vi "TIO SLIP Encode.vi"(2 "error in (no error)":errorcluster, 3 "String Input":string="\u00124VxÛ\u0000") -> (0 "error out":errorcluster, 1 "SLIP Output":string)   [LabVIEW 2017]
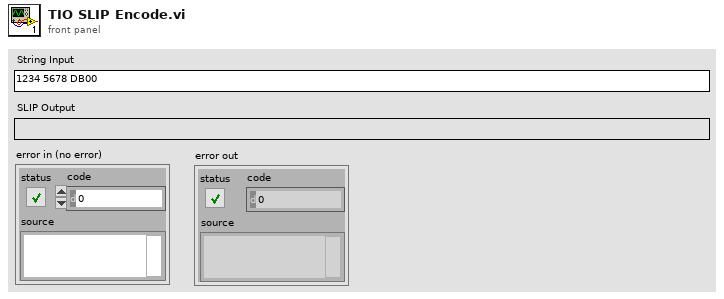
[diagram p1: front panel]
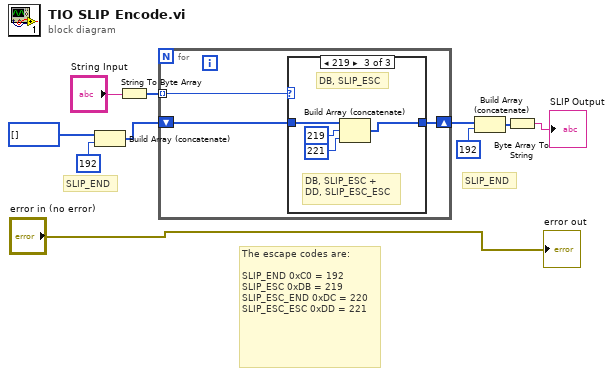
[diagram p0: block diagram]
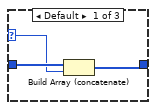
[diagram p2: hidden frame]
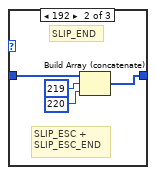
[diagram p3: hidden frame]
diagram:
  # "SLIP_END"
  # "SLIP_END"
  # "The escape codes are:\n\nSLIP_END\t0xC0 = 192\nSLIP_ESC\t0xDB = 219\nSLIP_ESC_END\t0xDC = 220\nSLIP_ESC_ESC\t0xDD = 221"
  n1 = Build Array (concatenate)(u8[] [] ("unsigned byte array"), u8 192) -> (w2:u8[])
  n2 = String To Byte Array(string="String Input") -> (unsigned byte array=w9:u8[])
  n3 = for {
    tunnel: w9 -> [w11] mode=indexing
    shift-right: [w12] -> w8
    shift-left: w2 -> [w13]
    n4 = case shown="219" w11 {
      selector: w11 -> [w15 _ _]
      tunnel: w13 -> [w16 w18 w24]
      tunnel: [w14 w17 w21] -> w12
      frame Default {
        n5 = Build Array (concatenate)(w16, w15) -> (w14:u8[])
      }
      frame 192 {
        # "SLIP_ESC + \nSLIP_ESC_END"
        # "SLIP_END"
        n6 = Build Array (concatenate)(w18, u8 219, u8 220) -> (w17:u8[])
      }
      frame 219 {
        # "DB, SLIP_ESC + \nDD, SLIP_ESC_ESC"
        # "DB, SLIP_ESC"
        n7 = Build Array (concatenate)(w24, u8 219, u8 221) -> (w21:u8[])
      }
    }
  }
  n8 = Build Array (concatenate)(w8, u8 192) -> (w5:u8[])
  n9 = Byte Array To String(unsigned byte array=w5) -> (string=→"SLIP Output":string)
  "error out" <- "error in (no error)"
